vi "ShutdownError.vi"(7 "Timeout":u32, 8 "error in (no error)":errorcluster, 10 "Watchdog Name":string, 11 "Expired":bool) -> (0 "error out":errorcluster)   [LabVIEW 2017, in "Pound.lvclass"]
uses:
  <vilib>/NI/Software Watchdog/Pound/Pound.lvclass
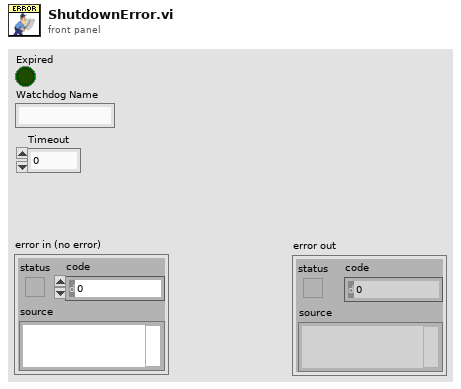
[diagram p1: front panel]
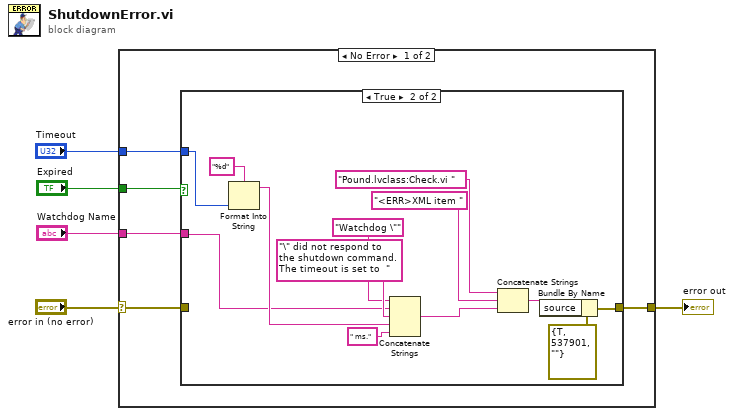
[diagram p0: block diagram]
diagram:
  n1 = case shown="No Error" "error in (no error)" {
    selector: "error in (no error)" -> [w8 w25]
    tunnel: [w7 w25] -> w4
    tunnel: "Expired" -> [w10 _]
    tunnel: "Watchdog Name" -> [w9 _]
    tunnel: "Timeout" -> [w6 _]
    frame No Error {
      n2 = case shown="True" w10 {
        tunnel: w9 -> [_ w12]
        tunnel: w8 -> [w11 _]
        tunnel: [w11 w14] -> w7
        tunnel: w6 -> [_ w13]
        frame False {
        }
        frame True {
          n3 = Format Into String(format string="%d", w13) -> (resulting string=w23:string)  [unwired: 2 in, 1 out]
          n4 = Concatenate Strings("Watchdog \"", w12, "\" did not respond to the shutdown command. The timeout is set to  ", w23, " ms." ("string")) -> (w21:string)
          n5 = Concatenate Strings("Pound.lvclass:Check.vi " ("string"), "<ERR>XML item " ("Format String"), w21) -> (w19:string)
          n6 = Bundle By Name(cluster=errorcluster {"status"=TRUE, "code"=537901, "source"=""} ("error in"), "source"=w19) -> (w14:errorcluster)
        }
      }
    }
    frame Error {
    }
  }
  "error out" <- w4
